vi "Init.vi"(8 "error in (no error)":errorcluster, 11 "Options":T1={"Login Path"="/login", "Identity Field"="_identity", "Password Field"="_password", "CSRF Field"="_csrf", "CSRF Token ID"="login", "Failure Path"="/login", "Logout Path"="/logout"}) -> (0 "error out":errorcluster, 3 "FormAuthentication out":refnum<class "FormAuthentication.lvclass">)   [LabVIEW 2020, in "HTTP Server.lvlib" / "FormAuthentication.lvclass"]
uses:
  FormAuthentication.lvclass
  Options.ctl
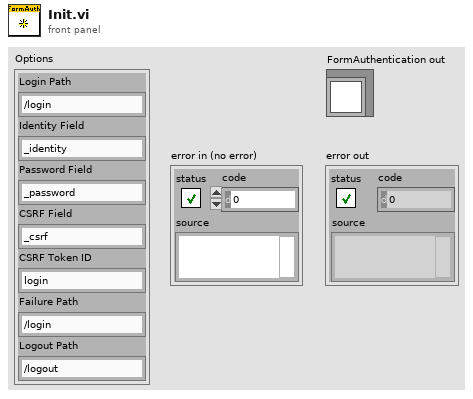
[diagram p1: front panel]
types:
  T1 = typedef "HTTP Server.lvlib/FormAuthentication.lvclass/Options.ctl" = cluster{"Login Path":string, "Identity Field":string, "Password Field":string, "CSRF Field":string, "CSRF Token ID":string, "Failure Path":string, "Logout Path":string}
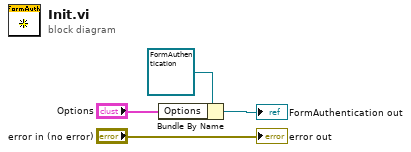
[diagram p0: block diagram]
diagram:
  n1 = Bundle By Name(cluster=refnum<class "FormAuthentication.lvclass"> refnum ("FormAuthentication out"), "Options"="Options") -> (→"FormAuthentication out":refnum<class "FormAuthentication.lvclass">)
  "error out" <- "error in (no error)"
